vi "ReciveThread.vi"() -> ()   [LabVIEW 2011]
uses:
  VIs/_USB_CAN_T_R_Unit_.ctl
  VIs/_USB_CAN_GLOBAL_.vi
  data/ControlCAN.dll
panel:
  in  "RcvLen":i32=48
  in  "Enable2":bool
  in  "Enable1":bool=TRUE
  in  "channels":i32=2
  in  "Scan time":u32=30
  in  "RFun":u16
  in  "DeviceInd":u32
  in  "type":u16(ring)=2 items=["USB-CAN"=2, "USB-CAN2.0"=3]
  in  "VCI_CAN_OBJ_R":u8[](array[numeric])=array[5000 elements]
  # "typedef struct _VCI_CAN_OBJ {\nBYTE ID[4];\nUINT TimeStamp;\nBYTE TimeFlag;\nBYTE SendType;\nBYTE RemoteFlag;\nBYTE ExternFlag;\nBYTE DataLen;\nBYTE Data[8];\nBYTE Reserved[3];} VCI_CAN_OBJ, *PVCI_CAN_OBJ;"
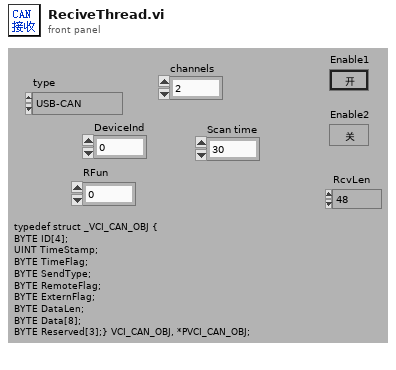
[diagram p1: front panel]
types:
  T1 = enum16{"open", "replace", "create", "open or create", "replace or create", "replace or create with confirmation"}
  T2 = typedef "_USB_CAN_T_R_Unit_.ctl" = cluster{"time":timestamp, "channel":u16, "TimeStamp":u32, "tr":enum16{"接收", "发送"}, "id":u32, "Type":enum16{"数据帧", "远程帧"}, "Format":enum16{"标准帧", "扩展帧"}, "len":u8, "data":u8[], "sysTime":u32}
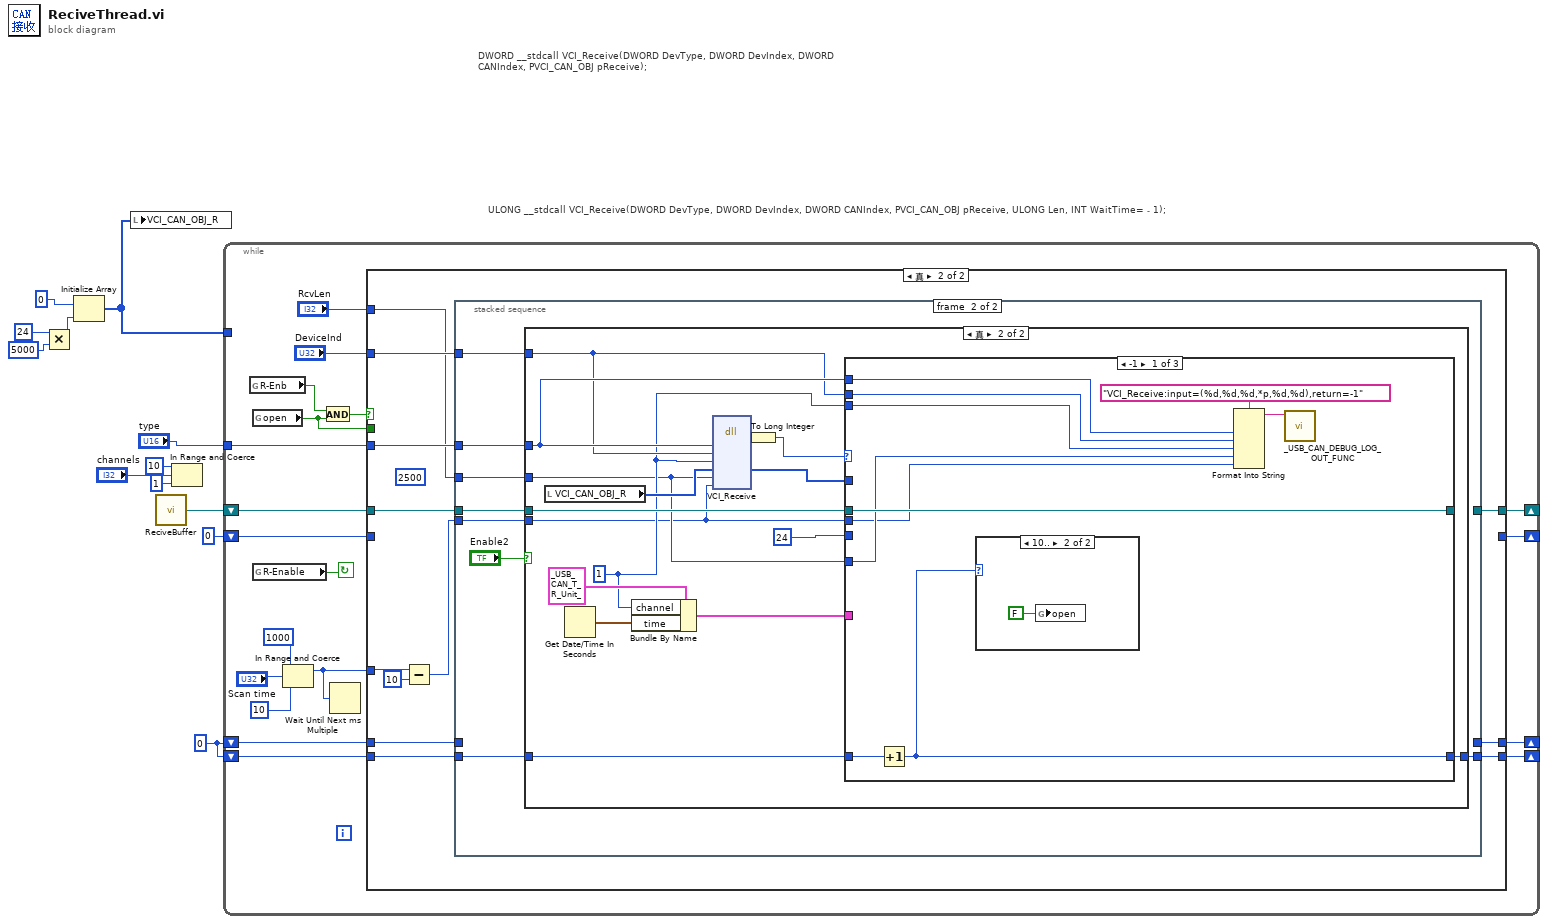
[diagram p0: block diagram]
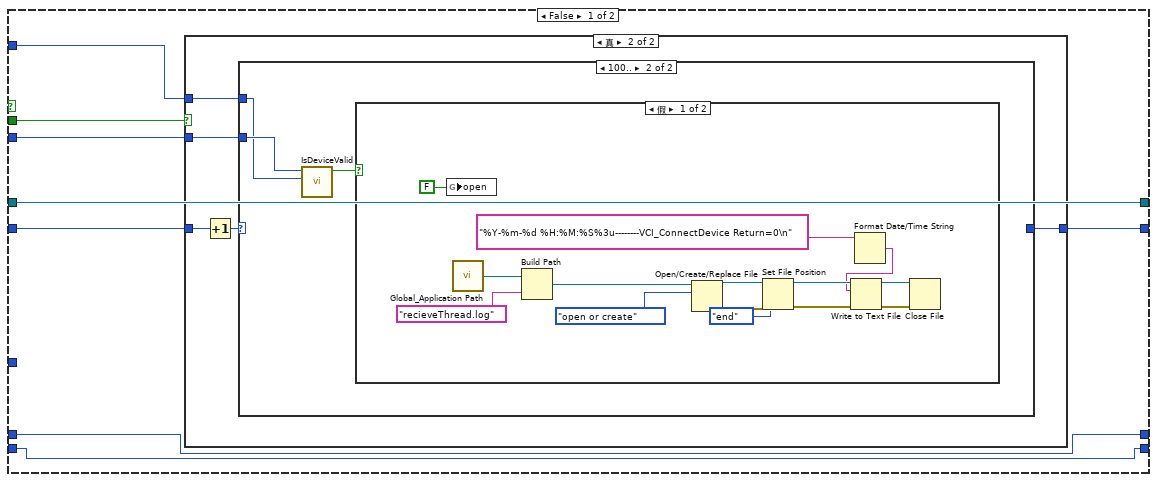
[diagram p2: hidden frame]
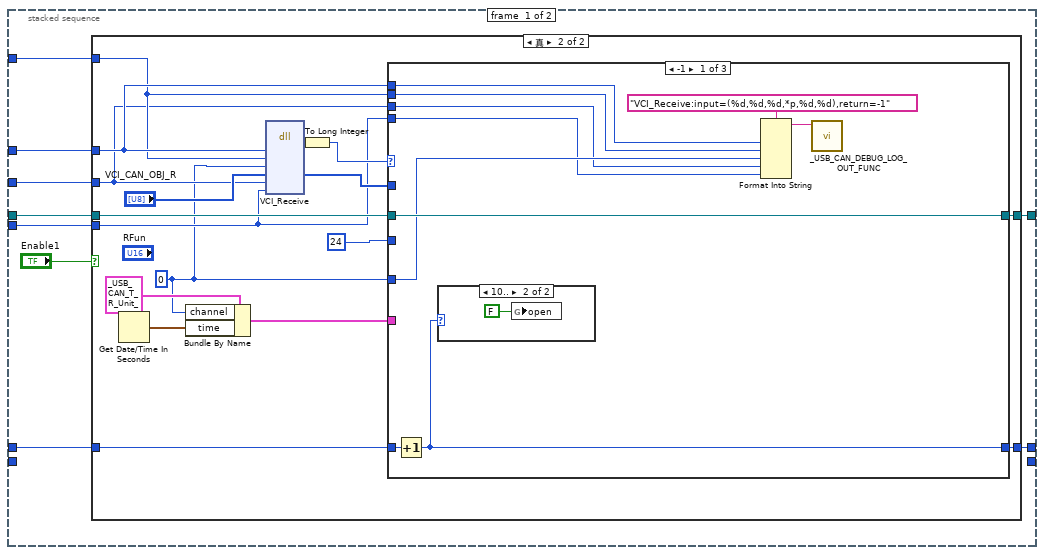
[diagram p6: hidden frame]
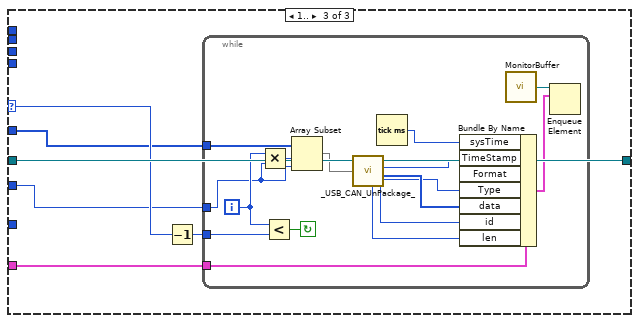
[diagram p10: hidden frame]
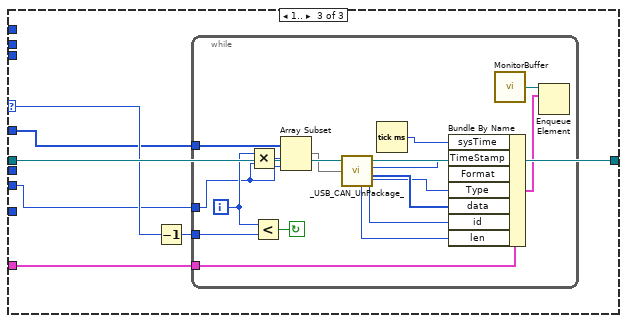
[diagram p14: hidden frame]
diagram:
  w1 = 0
  # "ULONG __stdcall VCI_Receive(DWORD DevType, DWORD DevIndex, DWORD CANIndex, PVCI_CAN_OBJ pReceive, ULONG Len, INT WaitTime=－1);"
  # "DWORD __stdcall VCI_Receive(DWORD DevType, DWORD DevIndex, DWORD\nCANIndex, PVCI_CAN_OBJ pReceive);"
  n1 = Multiply(x=24, y=5000 ("维数大小")) -> (x*y=w10:i32)
  n2 = Initialize Array(u8 0, w10) -> (w11:u8[])
  n3 = local write "VCI_CAN_OBJ_R"(w11) -> ()
  n4 = call "ReciveBuffer.vi"() -> ("VCI_USB_CAN_T_BUF_R"=w7:refnum<queue>)  [unwired: 1 in]
  n5 = In Range and Coerce(upper limit=10 ("上限"), x="channels", lower limit=1 ("下限")) -> ()  [unwired: 2 out]
  n6 = while {
    shift-right: [w30] -> _
    shift-left: w7 -> [w31]
    tunnel: "type" -> [w29]
    tunnel: w11 -> [_]
    shift-right: [w24] -> _
    shift-left: 0 -> [w25]
    shift-right: [w17] -> _
    shift-left: w1 -> [w18]
    shift-right: [w15] -> _
    shift-left: w1 -> [w16]
    stop <- w19 continue-if-true
    n7 = global read "_USB_CAN_GLOBAL_.vi" "R-Enb"() -> (w27:bool)
    n8 = global read "_USB_CAN_GLOBAL_.vi" "open"() -> (w26:bool)
    n9 = global read "_USB_CAN_GLOBAL_.vi" "R-Enable"() -> (w19:bool)
    n10 = In Range and Coerce(upper limit=u32 1000 ("上限"), x="Scan time", lower limit=u32 10 ("下限")) -> (coerced(x)=w13:u32)  [unwired: 1 out]
    n11 = And(x=w27, y=w26) -> (x .and. y?=w28:bool)
    n12 = Wait Until Next ms Multiple(millisecond multiple=w13) -> ()  [unwired: 1 out]
    n13 = case shown="真" w28 {
      tunnel: w29 -> [w35 w74]
      tunnel: w31 -> [w39 w73]
      tunnel: [w39 w72] -> w30
      tunnel: w26 -> [w38 _]
      tunnel: w25 -> [w37 _]
      tunnel: [w36 _] -> w24
      tunnel: "DeviceInd" -> [w34 w71]
      tunnel: w18 -> [w33 w70]
      tunnel: [w33 w69] -> w17
      tunnel: w16 -> [w32 w68]
      tunnel: [w32 w67] -> w15
      tunnel: w13 -> [_ w66]
      tunnel: "RcvLen" -> [_ w64]
      frame False {
        n14 = case shown="真" w38 {
          tunnel: w37 -> [_ w44]
          tunnel: [_ w42] -> w36
          tunnel: w35 -> [_ w41]
          tunnel: w34 -> [_ w40]
          frame False {
          }
          frame True {
            n15 = Increment(x=w44) -> (x+1=w43:i32)
            n16 = case shown="100.." w43 {
              selector: w43 -> [w45 _]
              tunnel: [w45 _] -> w42
              tunnel: w41 -> [_ w48]
              tunnel: w40 -> [_ w47]
              frame 0, Default {
              }
              frame 100.. {
                n17 = call "IsDeviceValid.vi"("DeviceInd"=w47, "type"=w48) -> ("Valid"=w46:bool)  [unwired: 8 in, 1 out]
                n18 = case shown="假" w46 {
                  frame False {
                    n19 = global write "_USB_CAN_GLOBAL_.vi" "open"(FALSE ("open")) -> ()
                    n20 = call "Global_Application Path.vi"() -> ("程序路径"=w51:path)  [unwired: 1 in]
                    n21 = Build Path(base path=w51, name or relative path="recieveThread.log" ("名称或相对路径")) -> (appended path=w60:path)
                    n22 = Open/Create/Replace File(file path (use dialog)=w60, operation (0:open)=T1."open or create" ("操作(0:open)")) -> (refnum out=w58:refnum<file>, error out=w57:errorcluster)  [unwired: 4 in, 1 out]
                    n23 = Set File Position(refnum=w58, from (0:start)=enum16{"start", "end", "current"}."end" ("自（0:起始）"), error in=w57) -> (refnum out=w55:refnum<file>, error out=w54:errorcluster)  [unwired: 1 in]
                    n24 = Format Date/Time String(time format string (%c)="%Y-%m-%d %H:%M:%S%3u--------VCI_ConnectDevice Return=0\n" ("时间格式字符串(%c)")) -> (date/time string=w49:string)  [unwired: 2 in]
                    n25 = Write to Text File(file (use dialog)=w55, text=w49, error in=w54) -> (refnum out=w52:refnum<file>, error out=w53:errorcluster)  [unwired: 1 in, 1 out]
                    n26 = Close File(refnum=w52, error in=w53) -> ()  [unwired: 2 out]
                  }
                  frame True {
                  }
                }
              }
            }
          }
        }
      }
      frame True {
        (unwired) u32 2500 ("Len")
        n27 = Subtract(x=w66, y=u32 10) -> (x-y=w63:u32)
        n28 = stacked-sequence {
          tunnel: w74 -> [w83 w144]
          tunnel: w73 -> [w82 w143]
          tunnel: [w81 _] -> w72
          tunnel: w71 -> [w80 w142]
          tunnel: w64 -> [w78 w140]
          tunnel: w63 -> [w77 w139]
          tunnel: w70 -> [w76 _]
          tunnel: [w75 _] -> w69
          tunnel: w68 -> [_ w138]
          tunnel: [_ w137] -> w67
          frame #0 {
            n29 = case shown="真" "Enable1" {
              tunnel: w83 -> [_ w89]
              tunnel: w82 -> [w84 w101]
              tunnel: [w84 w100] -> w81
              tunnel: w80 -> [_ w88]
              tunnel: w78 -> [_ w87]
              tunnel: w77 -> [_ w86]
              tunnel: w76 -> [_ w93]
              tunnel: [_ w92] -> w75
              frame False {
              }
              frame True {
                w85 = 0
                n30 = Get Date/Time In Seconds() -> (seconds since 1Jan1904=w96:timestamp)
                n31 = Bundle By Name(cluster=T2 {"time"=timestamp(0 s since 1904-01-01), "channel"=0, "TimeStamp"=0, "tr"=enum."接收", "id"=0, "Type"=enum."数据帧", "Format"=enum."标准帧", "len"=0, "data"=[], "sysTime"=0} ("TR_Unit"), "channel"=w85, "time"=w96) -> (w95:T2)
                n32 = dll-call lib="PTH1dabs CDocuments and Settings\nAdministrator桌面[CODE]USBCANTOOL2.04dataControlCAN.dll" fn="VCI_Receive"("DeviceType"=w89, "DeviceInd"=w88, "CANInd"=w85, "pReceive"="VCI_CAN_OBJ_R", "Len"=w87, "WaitTime"=w86) -> ("返回类型"=w90:u32, "pReceive"=w99:u8[])  [unwired: 8 in, 2 out]
                n33 = To Long Integer(number=w90) -> (32bit integer=w91:i32)
                n34 = case shown="-1" w91 {
                  selector: w91 -> [_ _ w118]
                  tunnel: w99 -> [_ _ w117]
                  tunnel: w101 -> [w111 w113 w119]
                  tunnel: [w111 w113 w119] -> w100
                  tunnel: 24 ("y") -> [_ _ w115]
                  tunnel: w95 -> [_ _ w114]
                  tunnel: w93 -> [w110 _ _]
                  tunnel: [w109 _ _] -> w92
                  tunnel: w89 -> [w107 _ _]
                  tunnel: w88 -> [w106 _ _]
                  tunnel: w87 -> [w104 _ _]
                  tunnel: w86 -> [w103 _ _]
                  tunnel: w85 -> [w105 _ _]
                  frame -1 {
                    n35 = Increment(x=w110) -> (x+1=w109:i32)
                    n36 = case shown="10.." w109 {
                      frame 0, Default {
                      }
                      frame 10.. {
                        n37 = global write "_USB_CAN_GLOBAL_.vi" "open"(FALSE ("open")) -> ()
                      }
                    }
                    n38 = Format Into String(format string="VCI_Receive:input=(%d,%d,%d,*p,%d,%d),return=-1", w107, w106, w105, w104, w103) -> (resulting string=w102:string)  [unwired: 2 in, 1 out]
                    n39 = call "_USB_CAN_DEBUG_LOG_OUT_FUNC.vi"("Info"=w102) -> ()  [unwired: 11 in]
                  }
                  frame 0, Default {
                  }
                  frame 1.. {
                    n40 = Decrement(x=w118) -> (x-1=w116:i32)
                    n41 = while {
                      tunnel: w116 -> [w134]
                      tunnel: w117 -> [w133]
                      tunnel: w114 -> [w130]
                      tunnel: w115 -> [w122]
                      i -> [w132]
                      stop <- w135 continue-if-true
                      n42 = Multiply(x=w132, y=w122) -> (x*y=w136:i32)
                      n43 = Less?(x=w132, y=w134) -> (x < y?=w135:bool)
                      n44 = Array Subset(array=w133, index=w136, length=w122) -> (w131:u8[])
                      n45 = call "_USB_CAN_UnPackage_.vi"("source"=w131) -> ("length"=w126:i32, "Type"=w123:enum16{"数据帧", "远程帧"}, "Format"=w124:enum16{"标准帧", "扩展帧"}, "TimeStamp"=w121:u32, "data"=w129:u8[], "ID"=w125:u32)
                      n46 = Tick Count (ms)() -> (millisecond timer value=w120:u32)
                      n47 = Bundle By Name(cluster=w130, "sysTime"=w120, "TimeStamp"=w121, "Format"=w124, "Type"=w123, "data"=w129, "id"=w125, "len"=w126) -> (w127:T2)
                      n48 = call "MonitorBuffer.vi"() -> ("USB_CAN_M_BUF"=w128:refnum<queue>)  [unwired: 1 in]
                      n49 = Enqueue Element(queue=w128, element=w127) -> ()  [unwired: 2 in, 3 out]
                    }
                  }
                }
              }
            }
          }
          frame #1 {
            n50 = case shown="真" "Enable2" {
              tunnel: w144 -> [_ w149]
              tunnel: w143 -> [_ w160]
              tunnel: w142 -> [_ w148]
              tunnel: w140 -> [_ w146]
              tunnel: w139 -> [_ w145]
              tunnel: w138 -> [_ w153]
              tunnel: [_ w152] -> w137
              frame False {
              }
              frame True {
                w147 = 1
                n51 = local read "VCI_CAN_OBJ_R"() -> (w155:u8[])
                n52 = Get Date/Time In Seconds() -> (seconds since 1Jan1904=w157:timestamp)
                n53 = Bundle By Name(cluster=T2 {"time"=timestamp(0 s since 1904-01-01), "channel"=0, "TimeStamp"=0, "tr"=enum."接收", "id"=0, "Type"=enum."数据帧", "Format"=enum."标准帧", "len"=0, "data"=[], "sysTime"=0} ("TR_Unit"), "channel"=w147, "time"=w157) -> (w156:T2)
                n54 = dll-call lib="PTH1dabs CDocuments and Settings\nAdministrator桌面[CODE]USBCANTOOL2.04dataControlCAN.dll" fn="VCI_Receive"("DeviceType"=w149, "DeviceInd"=w148, "CANInd"=w147, "pReceive"=w155, "Len"=w146, "WaitTime"=w145) -> ("返回类型"=w150:u32, "pReceive"=w159:u8[])  [unwired: 8 in, 2 out]
                n55 = To Long Integer(number=w150) -> (32bit integer=w151:i32)
                n56 = case shown="-1" w151 {
                  selector: w151 -> [_ _ w177]
                  tunnel: w159 -> [_ _ w176]
                  tunnel: w160 -> [w170 w172 w178]
                  tunnel: [w170 w172 w178] -> _
                  tunnel: 24 ("y") -> [_ _ w174]
                  tunnel: w156 -> [_ _ w173]
                  tunnel: w153 -> [w169 _ _]
                  tunnel: [w168 _ _] -> w152
                  tunnel: w149 -> [w165 _ _]
                  tunnel: w148 -> [w164 _ _]
                  tunnel: w147 -> [w163 _ _]
                  tunnel: w146 -> [w162 _ _]
                  tunnel: w145 -> [w161 _ _]
                  frame -1 {
                    n57 = Increment(x=w169) -> (x+1=w168:i32)
                    n58 = case shown="10.." w168 {
                      frame 0, Default {
                      }
                      frame 10.. {
                        n59 = global write "_USB_CAN_GLOBAL_.vi" "open"(FALSE ("open")) -> ()
                      }
                    }
                    n60 = Format Into String(format string="VCI_Receive:input=(%d,%d,%d,*p,%d,%d),return=-1", w165, w164, w163, w162, w161) -> (resulting string=w166:string)  [unwired: 2 in, 1 out]
                    n61 = call "_USB_CAN_DEBUG_LOG_OUT_FUNC.vi"("Info"=w166) -> ()  [unwired: 11 in]
                  }
                  frame 0, Default {
                  }
                  frame 1.. {
                    n62 = Decrement(x=w177) -> (x-1=w175:i32)
                    n63 = while {
                      tunnel: w175 -> [w193]
                      tunnel: w176 -> [w192]
                      tunnel: w173 -> [w189]
                      tunnel: w174 -> [w181]
                      i -> [w191]
                      stop <- w194 continue-if-true
                      n64 = Multiply(x=w191, y=w181) -> (x*y=w195:i32)
                      n65 = Less?(x=w191, y=w193) -> (x < y?=w194:bool)
                      n66 = Array Subset(array=w192, index=w195, length=w181) -> (w190:u8[])
                      n67 = call "_USB_CAN_UnPackage_.vi"("source"=w190) -> ("length"=w185:i32, "Type"=w182:enum16{"数据帧", "远程帧"}, "Format"=w183:enum16{"标准帧", "扩展帧"}, "TimeStamp"=w180:u32, "data"=w188:u8[], "ID"=w184:u32)
                      n68 = Tick Count (ms)() -> (millisecond timer value=w179:u32)
                      n69 = Bundle By Name(cluster=w189, "sysTime"=w179, "TimeStamp"=w180, "Format"=w183, "Type"=w182, "data"=w188, "id"=w184, "len"=w185) -> (w186:T2)
                      n70 = call "MonitorBuffer.vi"() -> ("USB_CAN_M_BUF"=w187:refnum<queue>)  [unwired: 1 in]
                      n71 = Enqueue Element(queue=w187, element=w186) -> ()  [unwired: 2 in, 3 out]
                    }
                  }
                }
              }
            }
          }
        }
      }
    }
  }
